vi "Do.vi"(8 "error in":errorcluster, 10 "Actor in":refnum<class "Actor.lvclass">, 11 "Toggle USB MSG":refnum<class "Toggle USB MSG.lvclass">) -> (0 "error out":errorcluster, 2 "Actor out":refnum<class "Actor.lvclass">)   [LabVIEW 2017, in "Controller.lvlib" / "Toggle USB MSG.lvclass"]
doc: "(<B>Filename</B>: Actor Framework.lvlib:Message.lvclass:Do.vi)\n\nDefines what a message does when it is received by an actor. Generally, a message instructs an actor to invoke one of its methods. By default, this method does nothing. A child class must override it to define behavior. Create a child class by using the Actor Framework Message Maker dialog box."
uses:
  Toggle USB MSG.lvclass
  U:/sw_repo/For Builds/Nicholas/Controller/Messages/Generic Boolean MSG/Generic Boolean Message.lvclass
  <vilib>/ActorFramework/Actor/Actor.lvclass
  Generic Boolean MSG/Generic Boolean Message.lvclass/Generic Boolean Message.ctl
  gController.lvclass
  C:/Program Files (x86)/National Instruments/LabVIEW 2017/vi.lib/ActorFramework/Actor/Actor.lvclass
  C:/Program Files (x86)/National Instruments/LabVIEW 2017/vi.lib/MSR Consulting, LLC/General Reuse/SuperActor/SuperActor.lvclass
  <vilib>/MSR Consulting, LLC/General Reuse/SuperActor/SuperActor.lvclass/SuperActor.ctl
  Global FPGA DO.ctl
  Generic Boolean MSG/Read Bool.vi
  <vilib>/MSR Consulting, LLC/General Reuse/SuperActor/Read Log Session.vi
  Global DO.vi
  <vilib>/rvi/errors/niLvFpgaAdjustHostInterfaceError.vi
  <vilib>/Utility/error.llb/Error Cluster From Error Code.vi
  FPGA Ref.ctl
  <vilib>/rvi/interface/nirviReadWriteControl/nirviReadWriteControl.xnode
  FPGA Bitfiles/server.lvbitx
  <vilib>/MSR Consulting, LLC/General Reuse/Session APIs/_Session Fwk/Session - Root.lvclass
  <vilib>/MSR Consulting, LLC/General Reuse/Session APIs/Session Log/System Log.lvclass
  NiFpgaLv.dll
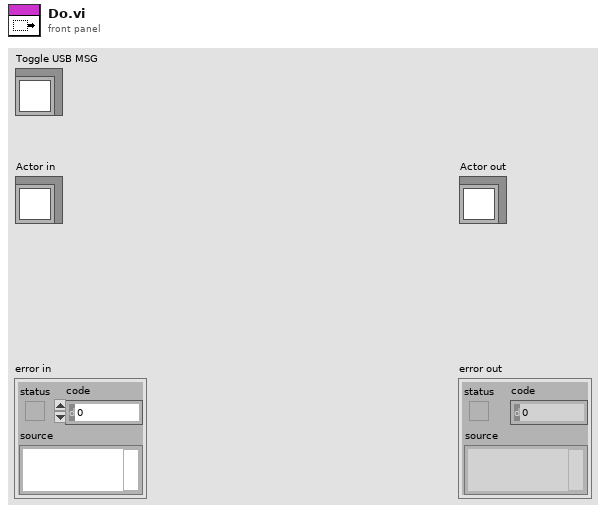
[diagram p1: front panel]
types:
  T1 = typedef "Global FPGA DO.ctl" = enum16{"pas_laser_relay_1", "pas_heater_1", "pas_heater_2", "pas_laser_relay_2", "pas_spk_enable_1", "pas_spk_enable_2", "hanbay_pos", "fan_enable", "crd_laser_enable", "crd_heater_enable", "vacuum_pump", "ac_spare", "uv_enable", "solenoid_1", "solenoid_2", "spare_dc_relay_1", "usb_hub_relay", "spare_dc_relay_2", "fp_aux_1", "fp_aux_2"}
  T2 = typedef "Session - Root.lvclass/Session Handle.ctl" = refnum<data-value>
  T3 = typedef "FPGA Ref.ctl" = refnum<k20>
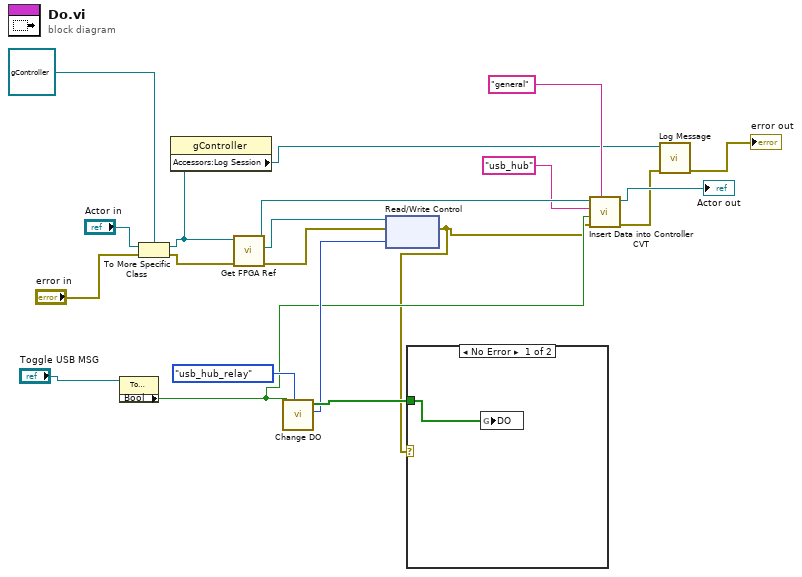
[diagram p0: block diagram]
diagram:
  n1 = property class="Toggle USB MSG"(reference="Toggle USB MSG") -> ("Bool"=w6:bool)  [unwired: 1 in, 2 out]
  n2 = To More Specific Class(target class=refnum<class "gController.lvclass"> refnum ("Controller.lvlib:gController"), reference="Actor in", error in="error in") -> (specific class reference=w4:refnum<class "gController.lvclass">, error out=w14:errorcluster)
  n3 = property class="gController"(reference=w4) -> ("Accessors:Log Session"=w3:T2)  [unwired: 1 in, 2 out]
  n4 = call "Get FPGA Ref.vi"("error in (no error)"=w14, "Actor In"=w4) -> ("error out"=w11:errorcluster, "FPGA Ref"=w13:T3, "Actor Out"=w9:refnum<class "Actor.lvclass">)  [unwired: 7 in]
  n5 = call "Change DO.vi"("DO"=Global_FPGA_DO."usb_hub_relay", "val_in"=w6) -> ("DO Long Out"=w12:u32, "DO Out"=w16:bool[])  [unwired: 8 in]
  n6 = xnode "Read/Write Control"("FPGA VI Reference In"=w13, "error in"=w11, "DO"=w12) -> ("error out"=w5:errorcluster)  [unwired: 1 out]
  n7 = case shown="No Error" w5 {
    tunnel: w16 -> [w21 _]
    frame No Error {
      n8 = global write "Global DO.vi" "DO"(w21) -> ()
    }
    frame Error {
    }
  }
  n9 = call "Insert Data into Controller CVT.vi"("Group"="general", "error in"=w5, "Data"=w6, "tag"="usb_hub", "Actor in"=w9) -> ("error out"=w2:errorcluster, "Actor Out"=→"Actor out":refnum<class "Actor.lvclass">)  [unwired: 5 in]
  n10 = call <vilib>:"Log Message.vi"("error in"=w2, "session in"=w3) -> ("error out"=→"error out":errorcluster)  [unwired: 8 in, 1 out]
